vi "ClassicEventDrivenVI-unfinished.vi"() -> ()   [LabVIEW 2014]
panel:
  in  "stop":bool
  out "What happened?":string
  in  "Button 2":bool
  in  "Button 1":bool
  in  "Numeric":dbl
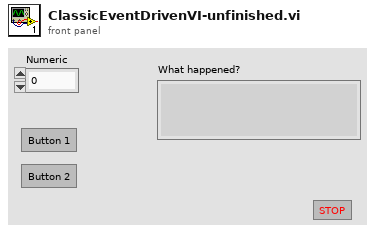
[diagram p1: front panel]
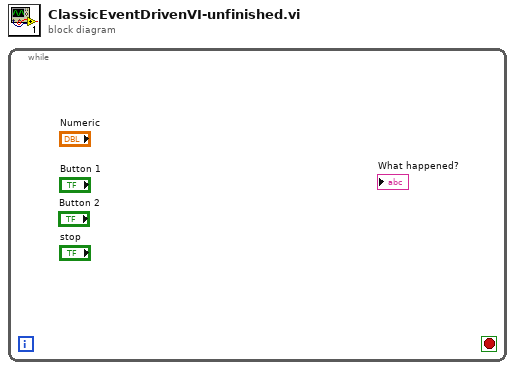
[diagram p0: block diagram]
diagram:
  n1 = while {
    stop <- _ stop-if-true
  }
